vi "text파일로 저장되어 있는 위도경도 데이터 k, k+1점 분리 & 벡터계산.vi"() -> ()   [LabVIEW 2016]
uses:
  DLL/distance_of_P1toP2.dll
  DLL/bearingP1toP2.dll
panel:
  in  "?":i32=1
  out "Distance (m)":dbl format="%#.6g"
  out "Bearing angle (deg)":u16
  out "(k+1)번째":i32
  out "k번째":i32
  out "Longitude 2":string
  out "Latitude 2":string
  out "Latitude 1":string
  out "Longitude 1":string
  in  "파일(대화 상자 사용)":path=path "C:/Users/user/Desktop/작업중인 모든 Vi, dll파일 모음/Global Mapping Data.txt"
  # "번째 경유점"
  # "번째 경유점"
  # "k번째 경유점"
  # "Bearing\n angle"
  # "Distance"
  # "m"
  # "deg"
  # "="
  # "="
  # "k  ="
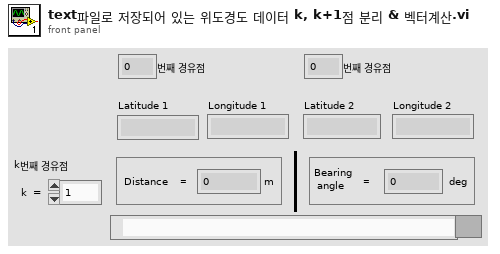
[diagram p1: front panel]
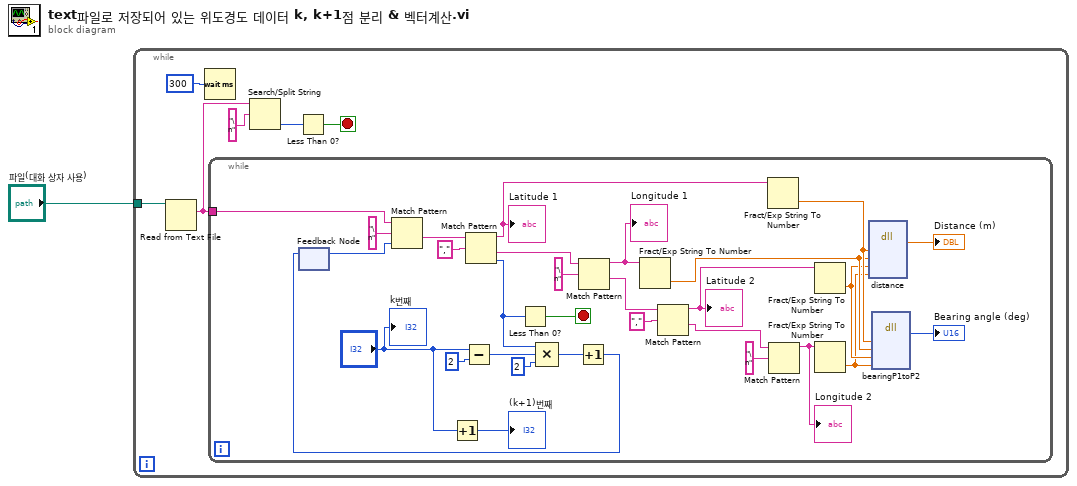
[diagram p0: block diagram]
diagram:
  n1 = while {
    tunnel: "파일(대화 상자 사용)" -> [w3]
    stop <- w6 stop-if-true
    n2 = Read from Text File(file (use dialog)=w3) -> (text=w2:string)  [unwired: 3 in, 3 out]
    n3 = Wait (ms)(milliseconds to wait=u32 300 ("대기 시간 (ms)")) -> ()  [unwired: 1 out]
    n4 = while {
      tunnel: w2 -> [w32]
      stop <- w37 stop-if-true
      n5 = feedback #1() -> (w22:i32)  [unwired: 1 in]
      n6 = Match Pattern(string=w32, regular expression="\n" ("정규식"), offset (0)=w22) -> (after substring=w31:string)  [unwired: 3 out]
      n7 = Increment(x="?") -> (x+1=→"(k+1)번째":i32)
      n8 = Subtract(x="?", y=2) -> (x-y=w10:i32)
      n9 = Match Pattern(string=w31, regular expression="," ("search string/char (-)")) -> (before substring=w21:string, after substring=w35:string, offset past match=w25:i32)  [unwired: 1 in, 1 out]
      "Latitude 1" <- w21
      n10 = Less Than 0?(x=w25) -> (x < 0?=w37:bool)
      n11 = Compound Arithmetic op=MULTIPLY(w25, w10, 2 ("값")) -> (w24:i32)
      n12 = Increment(x=w24) -> (x+1=w23:i32)
      n13 = feedback-in #1(w23) -> ()
      n14 = Match Pattern(string=w35, regular expression="\n" ("정규식")) -> (before substring=w20:string, after substring=w26:string)  [unwired: 1 in, 2 out]
      "Longitude 1" <- w20
      n15 = Fract/Exp String To Number(string=w20) -> (number=w14:dbl)  [unwired: 3 in, 1 out]
      n16 = Match Pattern(string=w26, regular expression="," ("search string/char (-)")) -> (before substring=w19:string, after substring=w28:string)  [unwired: 1 in, 2 out]
      "Latitude 2" <- w19
      n17 = Fract/Exp String To Number(string=w21) -> (number=w15:dbl)  [unwired: 3 in, 1 out]
      n18 = Match Pattern(string=w28, regular expression="\n" ("정규식")) -> (before substring=w18:string)  [unwired: 1 in, 3 out]
      "Longitude 2" <- w18
      n19 = Fract/Exp String To Number(string=w19) -> (number=w13:dbl)  [unwired: 3 in, 1 out]
      n20 = Fract/Exp String To Number(string=w18) -> (number=w12:dbl)  [unwired: 3 in, 1 out]
      n21 = dll-call lib="PTH2abs CUsersuserDesktop[Github]_GPS Teamlabview_program(ììì¤ì¸ ëª¨ë  Vi, dllíì¼ ëª¨ìì ì²´íë¡ê·¸ë¨DLLdistance_of_P1toP2.dll" fn="distance" label="사이 거리"("P1_latitude"=w15, "P1_longitude"=w14, "P2_latitude"=w13, "P2_longitude"=w12) -> ("반환 타입"=→"Distance (m)":dbl)  [unwired: 7 in, 2 out]
      n22 = dll-call lib="PTH2abs CUsersuserDesktop[Github]_GPS Teamlabview_program(ììì¤ì¸ ëª¨ë  Vi, dllíì¼ ëª¨ìì ì²´íë¡ê·¸ë¨DLLbearingP1toP2.dll" fn="bearingP1toP2" label="방향각"("P1_latitude"=w15, "P1_longitude"=w14, "P2_latitude"=w13, "P2_longitude"=w12) -> ("반환 타입"=→"Bearing angle (deg)":u16)  [unwired: 7 in, 2 out]
      "k번째" <- "?"
    }
    n23 = Search/Split String(string=w2, search string/char (-)="\n") -> (offset of match=w5:i32)  [unwired: 3 out]
    n24 = Less Than 0?(x=w5) -> (x < 0?=w6:bool)
  }
